vi "save configuration file.vi"() -> ()   [LabVIEW 2016]
uses:
  <vilib>/Utility/config.llb/NI_LVConfig.lvlib
panel:
  in  "Write Ini":bool
  in  "Read Ini":bool
  in  "Path":path=path "C:/Users/CWEDD/Documents/LabVIEW Data/Waterloo DAQ/config files/DAQ Setup Config.ini"
  out "error out":errorcluster
  in  "error in (no error)":errorcluster
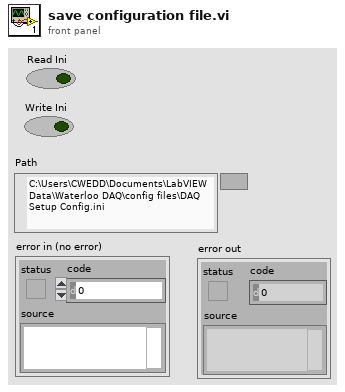
[diagram p1: front panel]
types:
  T1 = typedef "NI_LVConfig.lvlib/Config Data RefNum.ctl" = refnum<k1>
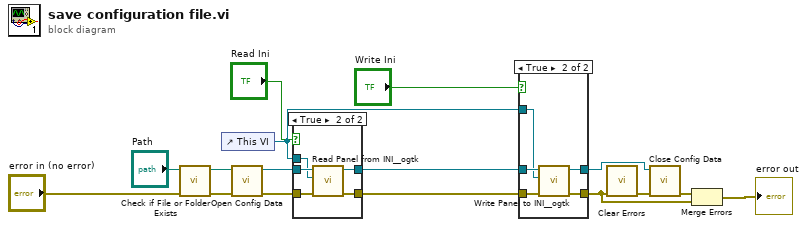
[diagram p0: block diagram]
diagram:
  n1 = call <vilib>:"Check if File or Folder Exists.vi"("error in (no error)"="error in (no error)", "path"="Path") -> ("error out"=w12:errorcluster, "dup path"=w13:path)  [unwired: 7 in, 1 out]
  n2 = control-ref of="This VI"() -> (w4:refnum<vi>)
  n3 = call <vilib>:"Open Config Data.vi"("error in (no error)"=w12, "configuration file path"=w13) -> ("error out"=w10:errorcluster, "refnum"=w11:T1)  [unwired: 7 in, 1 out]
  n4 = case shown="True" "Read Ini" {
    tunnel: w11 -> [w18 w23]
    tunnel: w10 -> [w17 w22]
    tunnel: w4 -> [_ w21]
    tunnel: [w17 w20] -> w5
    tunnel: [w18 w19] -> w6
    frame False {
    }
    frame True {
      n5 = call <userlib>:"Read Panel from INI__ogtk.vi"("error in (no error)"=w22, "VI ref"=w21, "refnum"=w23) -> ("error out"=w20:errorcluster, "refnum out"=w19:T1)  [unwired: 7 in]
    }
  }
  n6 = case shown="True" "Write Ini" {
    tunnel: w6 -> [w25 w30]
    tunnel: w5 -> [w24 w29]
    tunnel: w4 -> [_ w28]
    tunnel: [w25 w27] -> w3
    tunnel: [w24 w26] -> w2
    frame False {
    }
    frame True {
      n7 = call <userlib>:"Write Panel to INI__ogtk.vi"("error in (no error)"=w29, "VI ref"=w28, "refnum"=w30) -> ("error out"=w26:errorcluster, "refnum out"=w27:T1)  [unwired: 7 in]
    }
  }
  n8 = call <vilib>:"Clear Errors.vi"("error in (no error)"=w2) -> ("error out"=w9:errorcluster)  [unwired: 5 in, 1 out]
  n9 = call <vilib>:"Close Config Data.vi"("error in (no error)"=w9, "refnum"=w3) -> ("error out"=w8:errorcluster)  [unwired: 8 in, 1 out]
  n10 = Merge Errors(w8, w2) -> (→"error out":errorcluster)
